vi "AH Bridge Check Calibration and Re-Cal.vi"(8 "error in (no error)":errorcluster {"code" format="%.0x"}, 11 "VISA resource name":refnum<visa-resource-name>) -> (0 "error out":errorcluster {"code" format="%.0x"}, 2 "Calibration Out of Date":bool)   [LabVIEW 2025]
doc: "This VI checks the calibration date and recommends an internal calibration if the current date is greater than the due date for the internal calibration. This will eliminate the issue of various indicators (N, D) on the display that alert the user to the need for a recalibration.\n\nScott Hannahs - NHMFL\n<sth@magnet.fsu.edu>\nAuthor: Scott Hannahs <sth@magnet.fsu.edu>\n\nThis software is licensed for use under the “MIT License\"\nCopyright (c) 2025 Scott Hannahs, sth@sth@magnet.sthnet.net\n\nPermission is hereby granted, free of charge, to any person obtaining a copy of this software and associated documentation files (the \"Software\"), to deal in the Software without restriction, including without limitation the rights to use, copy, modify, merge, publish, distribute, sublicense, and/or sell copies of the Software, and to permit persons to whom the Software is furnished to do so, subject to the following conditions: The above copyright notice and this permission notice shall be included in all copies or substantial portions of the Software.\n\nTHE SOFTWARE IS PROVIDED \"AS IS\", WITHOUT WARRANTY OF ANY KIND, EXPRESS OR IMPLIED, INCLUDING BUT NOT LIMITED TO THE WARRANTIES OF MERCHANTABILITY, FITNESS FOR A PARTICULAR PURPOSE AND NONINFRINGEMENT. IN NO EVENT SHALL THE AUTHORS OR COPYRIGHT HOLDERS BE LIABLE FOR ANY CLAIM, DAMAGES OR OTHER LIABILITY, WHETHER IN AN ACTION OF CONTRACT, TORT OR OTHERWISE, ARISING FROM, OUT OF OR IN CONNECTION WITH THE SOFTWARE OR THE USE OR OTHER DEALINGS IN THE SOFTWARE."
uses:
  <vilib>/Utility/miscctls.llb/LVDateTimeRec.ctl
panel:
  out "Done":bool
  out "Time Remaining":dbl format="%<%H:%M:%S>t"
  out "Message":string="The AH Capacitance Bridge internal calibration is more than 6 months out of date.  Unplug the inputs to the bridge and press update to calibrate.  \n\nThis process will take about 30 min for all ranges and frequencies."
  in  "Calibrate Button":bool
  in  "Cancel Button":bool
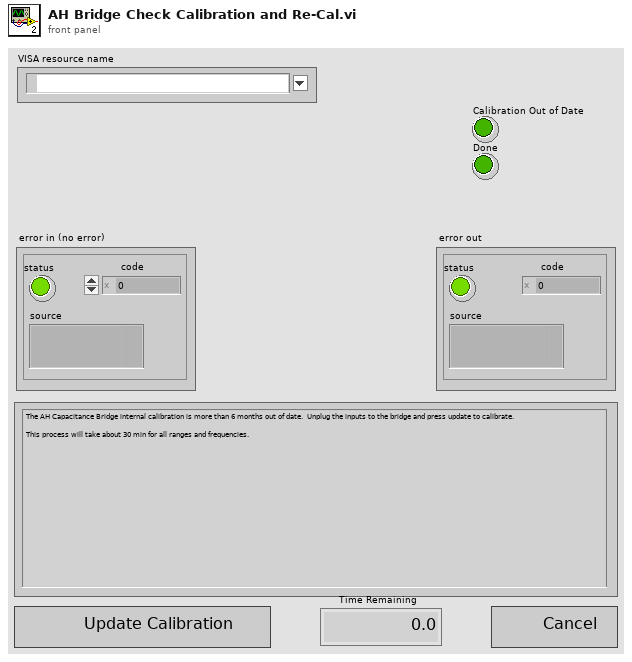
[diagram p1: front panel]
types:
  T1 = typedef "LVDateTimeRec.ctl" = cluster{"fractional second":dbl, "second":i32, "minute":i32, "hour":i32, "day of month":i32, "month":i32, "year":i32, "day of week":i32, "day of year":i32, "DST":i32}
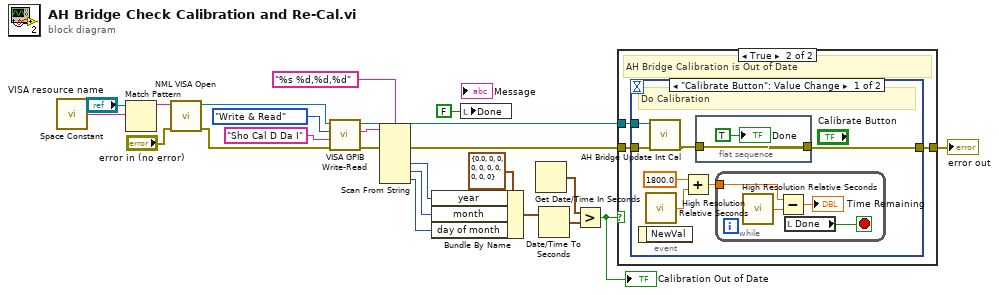
[diagram p0: block diagram]
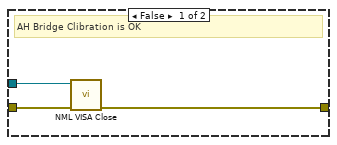
[diagram p2: hidden frame]
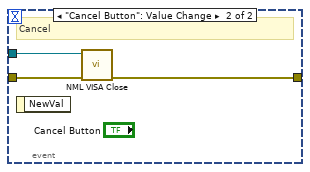
[diagram p3: hidden frame]
diagram:
  n1 = call <vilib>:"Space Constant.vi"() -> ("String"=w5:string)
  n2 = Match Pattern(string="VISA resource name", regular expression=w5) -> (before substring=w3:string)  [unwired: 1 in, 3 out]
  n3 = call "NML VISA Open.vi"("error in (no error)"="error in (no error)", "VISA resource name"=w3) -> ("error out"=w6:errorcluster, "VISA resource name out"=w7:refnum<visa-resource-name>)  [unwired: 8 in]
  n4 = call "VISA GPIB Write-Read.vi"("error in (no error)"=w6, "Command"="Sho Cal D Da I", "Action"=enum16{"Write", "Read", "Write & Read"}."Write & Read", "VISA resource name"=w7) -> ("error out"=w16:errorcluster, "String Returned"=w18:string, "dup VISA Session"=w10:refnum<visa-resource-name>)  [unwired: 4 in, 1 out]
  n5 = Scan From String(format string="%s %d,%d,%d", input string=w18, error in=w16) -> (error out=w9:errorcluster, output 2=w15:i32, output 3=w14:i32, output 4=w13:i32)  [unwired: 6 in, 2 out]
  n6 = Bundle By Name(cluster=T1 {"fractional second"=0.0, "second"=0, "minute"=0, "hour"=0, "day of month"=0, "month"=0, "year"=0, "day of week"=0, "day of year"=0, "DST"=0} ("date time rec"), "year"=w15, "month"=w14, "day of month"=w13) -> (w22:T1)
  n7 = local write "Done"(FALSE ("Done")) -> ()
  n8 = Get Date/Time In Seconds() -> (seconds since 1Jan1904=w12:timestamp)
  n9 = Date/Time To Seconds(2:w22) -> (0:w21:timestamp)  [unwired: 1 in]
  n10 = Greater?(x=w12, y=w21) -> (0:w11:bool)
  "Calibration Out of Date" <- w11
  n11 = case shown="True" w11 {
    tunnel: w10 -> [w26 w29]
    tunnel: w9 -> [w25 w28]
    tunnel: [w24 w27] -> w8
    frame False {
      # "AH Bridge Clibration is OK"
      n12 = call "NML VISA Close.vi"("Error In"=w25, "VISA resource name"=w26) -> ("Error Out"=w24:errorcluster)  [unwired: 9 in]
    }
    frame True {
      # "AH Bridge Calibration is Out of Date"
      n13 = event shown="[0] \"Calibrate Button\": Value Change" {
        selector: _ -> [_ _]
        dyn-events: _ -> [_ _]
        timeout: _ -> [_ _]
        tunnel: w29 -> [w35 w45]
        tunnel: w28 -> [w36 w44]
        tunnel: [w34 w43] -> w27
        event "Calibrate Button": Value Change {
          # "Do Calibration"
          n14 = event-data() -> ()  [unwired: 1 in, 1 out]
          n15 = call <vilib>:"High Resolution Relative Seconds.vi"() -> ("relative seconds"=w30:dbl)
          n16 = call "AH Bridge Update Int Cal.vi"("error in (no error)"=w36, "VISA resource name"=w35) -> ("error out"=w33:errorcluster)  [unwired: 6 in, 3 out]
          n17 = Add(x=1800.0, y=w30) -> (x+y=w31:dbl)
          n18 = flat-sequence {
            tunnel: [w42] -> w34
            tunnel: w33 -> [w42]
            frame #0 {
              "Done" <- TRUE ("Done")
            }
          }
          n19 = while {
            tunnel: w31 -> [w37]
            stop <- w38 stop-if-true
            n20 = call <vilib>:"High Resolution Relative Seconds.vi"() -> ("relative seconds"=w40:dbl)
            n21 = Subtract(x=w37, y=w40) -> (x-y=→"Time Remaining":dbl)
            n22 = local read "Done"() -> (w38:bool)
          }
        }
        event "Cancel Button": Value Change {
          # "Cancel"
          n23 = event-data() -> ()  [unwired: 1 in, 1 out]
          n24 = call "NML VISA Close.vi"("Error In"=w44, "VISA resource name"=w45) -> ("Error Out"=w43:errorcluster)  [unwired: 9 in]
        }
      }
    }
  }
  "error out" <- w8
